vi "mhk_Trap-Incremental_corrected_dA3.vi"() -> ()   [LabVIEW 2010]
uses:
  <vilib>/Analysis/2dsp.llb/Integral Method.ctl
  <vilib>/Analysis/8numeric.llb/1D Numeric Integration.vi
  <vilib>/Analysis/NI_AALPro.lvlib
panel:
  out "delta x":dbl=0.5
  in  "derivative method":u16(ring)=2 items=["2nd Order Central", "4th Order Central", "Forward", "Backward"]
  out "dX/dt":dbl[](array[numeric])=[-0.5475824447462729, -2.1420349857947287, 21.63314273516883, -24.672601291251752, -0.02751321193894931]
  out "function vector":dbl[](array[numeric])=[2.8782945992814364, 2.6045033769083, 1.5334858840109356, 12.35005725159535, 0.013756605969474655]
  out "accumulated da vector":dbl[](array[numeric])=[0.0, 1.3706994940474342, 2.405196809277243, 5.876082593178815, 8.96703605757002]
  out "Integral X":dbl[](array[numeric])=[0.0, 1.3706994940474342, 2.405196809277243, 5.876082593178815, 8.967036057570022]
  out "raw da vector":dbl[](array[numeric])=[0.0, 1.3706994940474342, 1.034497315229809, 3.4708857839015717, 3.090953464391206]
  out "function\nvector\nsize":i32=5
  out "da\nvector\nsize":i32=5
  out "1D integration\nresult":dbl=8.96703605757002 format="%0.5f"
  out "Running Integral Graph":cluster{"Lower limit \"a\"":dbl, dbl, dbl[][]}(graph)={"Lower limit \"a\""=2.8, 0.5, [[0.0, 1.3706994940474342, 1.034497315229809, 3.4708857839015717, 3.090953464391206], [0.0, 1.3706994940474342, 2.405196809277243, 5.876082593178815, 8.96703605757002], [0.0, 1.3706994940474342, 2.405196809277243, 5.876082593178815, 8.967036057570022]]}
  in  "Plot BG Color":bool
  out "Approx. Integral \nover entire range\ndone incrementally":dbl=8.96703605757002
  out "Approx. Integral \nover entire range\ndone en masse":dbl=8.967036057570022
  out "Function Graph":cluster{"Lower limit \"a\"":dbl, dbl, dbl[]}(graph)={"Lower limit \"a\""=2.8, 0.5, [2.8782945992814364, 2.6045033769083, 1.5334858840109356, 12.35005725159535, 0.013756605969474655]}
  in  "Divisions \"N\"":dbl=4.0
  in  "Upper limit \"b\"":dbl=4.8
  in  "Lower limit \"a\"":dbl=2.8
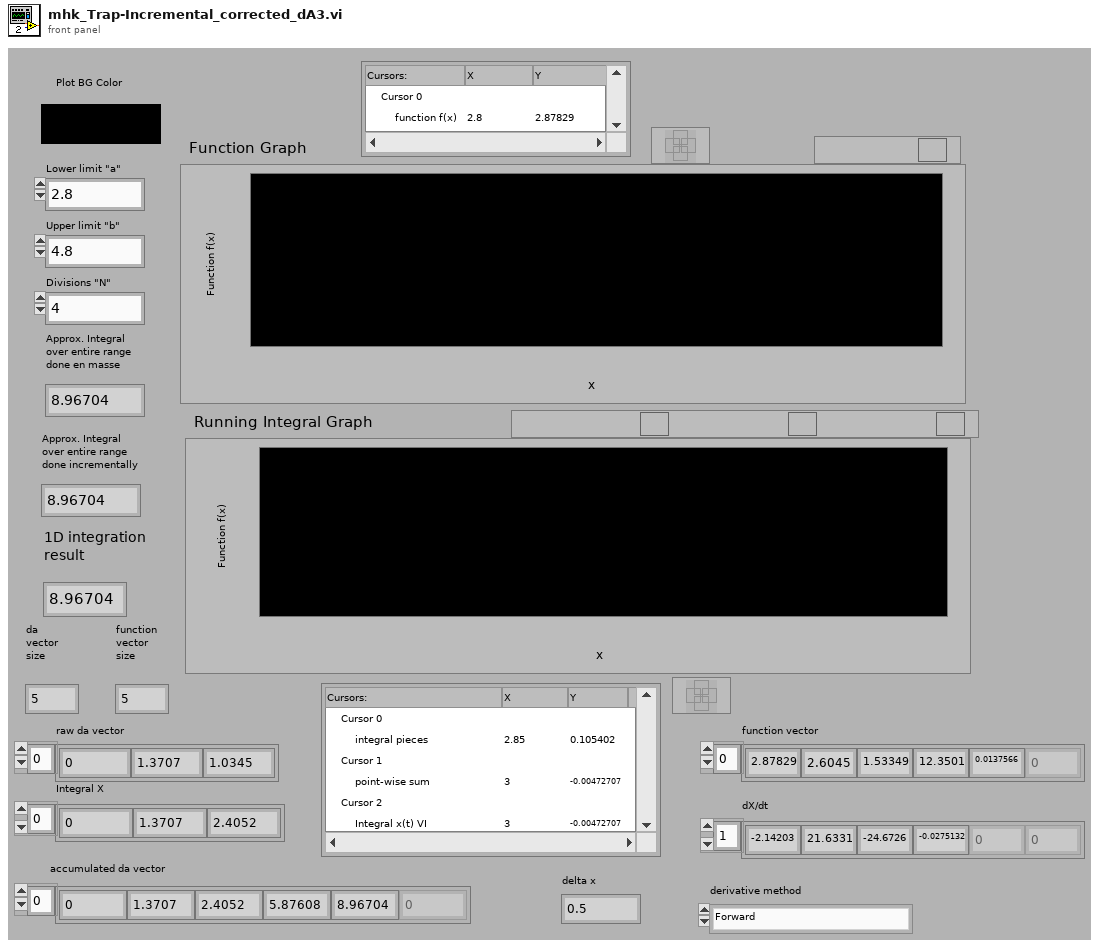
[diagram p1: front panel]
types:
  T1 = typedef "NI_AALPro.lvlib/Integral Method.ctl" = i32
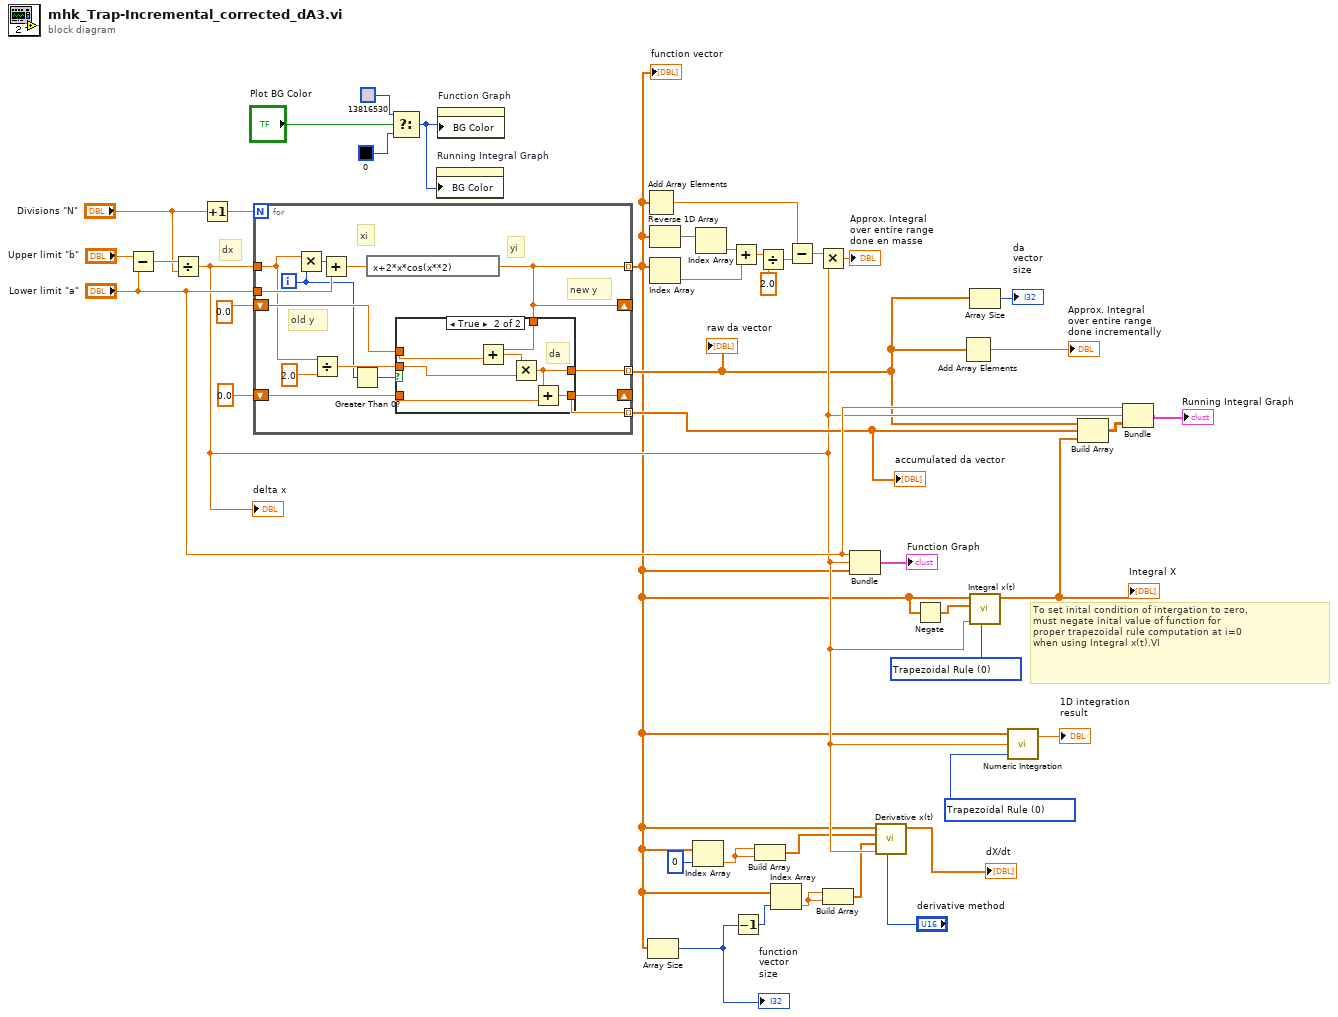
[diagram p0: block diagram]
diagram:
  w19 = T1 0 items=["Trapezoidal Rule", "Simpson's Rule", "Simpson's 3/8 Rule", "Bode Rule"] ("integration method")
  w21 = T1 0 items=["Trapezoidal Rule", "Simpson's Rule", "Simpson's 3/8 Rule", "Bode Rule"] ("integration method")
  # "To set inital condition of intergation to zero,\nmust negate inital value of function for \nproper trapezoidal rule computation at i=0 \nwhen using Integral x(t).VI"
  # "dx"
  n1 = Subtract(x="Upper limit \"b\"", y="Lower limit \"a\"") -> (x-y=w42:dbl)
  n2 = Divide(x=w42, y="Divisions \"N\"") -> (x/y=w18:dbl)
  "delta x" <- w18
  n3 = Increment(x="Divisions \"N\"") -> (x+1=w41:dbl)
  n4 = for {
    N: w41 -> [_]
    tunnel: w18 -> [w45]
    tunnel: "Lower limit \"a\"" -> [w55]
    tunnel: [w53] -> w3 mode=indexing
    shift-right: [w53] -> _
    shift-left: 0.0 -> [w52]
    tunnel: [w49] -> w12 mode=indexing
    shift-right: [w47] -> _
    shift-left: 0.0 -> [w48]
    tunnel: [w47] -> w23 mode=indexing
    i -> [w44]
    # "new y"
    # "old y"
    # "yi"
    # "xi"
    n5 = Multiply(x=w45, y=w44) -> (x*y=w56:dbl)
    n6 = Divide(x=w45, y=2.0) -> (x/y=w50:dbl)
    n7 = Add(x=w56, y=w55) -> (x+y=w54:dbl)
    n8 = Greater Than 0?(x=w44) -> (x > 0?=w46:bool)
    n9 = expression code="x+2*x*cos(x**2)"(w54) -> (w53:dbl)
    n10 = case shown="True" w46 {
      tunnel: w53 -> [_ w64]
      tunnel: w52 -> [_ w63]
      tunnel: w50 -> [_ w61]
      tunnel: [w57 w60] -> w49
      tunnel: w48 -> [w57 w59]
      tunnel: [w57 w58] -> w47
      frame False {
      }
      frame True {
        # "da"
        n11 = Add(x=w64, y=w63) -> (x+y=w62:dbl)
        n12 = Multiply(x=w62, y=w61) -> (x*y=w60:dbl)
        n13 = Add(x=w60, y=w59) -> (x+y=w58:dbl)
      }
    }
  }
  "raw da vector" <- w12
  "accumulated da vector" <- w23
  "function vector" <- w3
  n14 = Select(t=u32 13816530, s="Plot BG Color", f=u32 0) -> (s? t:f=w24:u32)
  n15 = property on="Running Integral Graph" class="WFGraph (strict)"("BG Color"=w24) -> ()  [unwired: 2 in, 2 out]
  n16 = property on="Function Graph" class="WFGraph (strict)"("BG Color"=w24) -> ()  [unwired: 2 in, 2 out]
  n17 = Add Array Elements(numeric array=w3) -> (sum=w33:dbl)
  n18 = Array Size(array=w3) -> (size(s)=w5:i32)
  "function\nvector\nsize" <- w5
  n19 = Reverse 1D Array(array=w3) -> (reversed array=w39:dbl[])
  n20 = Index Array(array=w3) -> (element=w37:dbl)  [unwired: 1 in]
  n21 = Index Array(array=w3, index=0) -> (element=w7:dbl)
  n22 = Index Array(array=w39) -> (element=w38:dbl)  [unwired: 1 in]
  n23 = Add(x=w38, y=w37) -> (x+y=w36:dbl)
  n24 = Decrement(x=w5) -> (x-1=w4:i32)
  n25 = Build Array(w7, w7) -> (w6:dbl[])
  n26 = Divide(x=w36, y=2.0) -> (x/y=w34:dbl)
  n27 = Index Array(array=w3, index=w4) -> (element=w2:dbl)
  n28 = Subtract(x=w33, y=w34) -> (x-y=w32:dbl)
  n29 = Multiply(x=w32, y=w18) -> (x*y=→"Approx. Integral \nover entire range\ndone en masse":dbl)
  n30 = Build Array(w2, w2) -> (w1:dbl[])
  n31 = Bundle("Lower limit \"a\""="Lower limit \"a\"", w18, w3) -> (→"Function Graph":cluster{"Lower limit \"a\"":dbl, dbl, dbl[]})  [unwired: 1 in]
  n32 = call <vilib>:"Derivative x(t).vi"("method"="derivative method", "dt"=w18, "Final Condition"=w1, "Initial Condition"=w6, "X"=w3) -> ("dX/dt"=→"dX/dt":dbl[])  [unwired: 5 in, 1 out]
  n33 = Negate(x=w3) -> (-x=w11:dbl[])
  n34 = Add Array Elements(numeric array=w12) -> (sum=→"Approx. Integral \nover entire range\ndone incrementally":dbl)
  n35 = Array Size(array=w12) -> (size(s)=→"da\nvector\nsize":i32)
  n36 = call <vilib>:"Integral x(t).vi"("integration method"=w19, "dt"=w18, "Initial Condition"=w11, "X"=w3) -> ("Integral X"=w14:dbl[])  [unwired: 6 in, 1 out]
  "Integral X" <- w14
  n37 = call-poly <vilib>:"Numeric Integration.vi"("integration method"=w21, "dt"=w18, "Input Array"=w3) -> ("result"=→"1D integration\nresult":dbl)  [unwired: 1 out]
  n38 = Build Array(w12, w23, w14) -> (w22:dbl[][])
  n39 = Bundle("Lower limit \"a\""="Lower limit \"a\"", w18, w22) -> (→"Running Integral Graph":cluster{"Lower limit \"a\"":dbl, dbl, dbl[][]})  [unwired: 1 in]
